vi "Vessel Blowout.vi"(7 "Blowtime(ms)":u32=5000, 9 "Delay(ms)":u32) -> ()   [LabVIEW 2019]
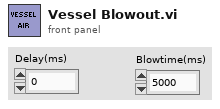
[diagram p1: front panel]
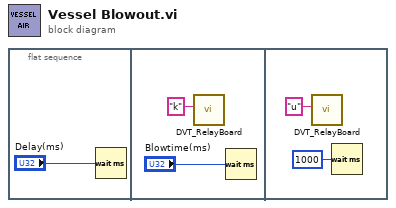
[diagram p0: block diagram]
diagram:
  n1 = flat-sequence {
    frame #0 {
      n2 = Wait (ms)(milliseconds to wait="Delay(ms)") -> ()  [unwired: 1 out]
    }
    frame #1 {
      n3 = call "DVT_RelayBoard.vi"("write buffer"="k") -> ()  [unwired: 3 in, 3 out]
      n4 = Wait (ms)(milliseconds to wait="Blowtime(ms)") -> ()  [unwired: 1 out]
    }
    frame #2 {
      n5 = call "DVT_RelayBoard.vi"("write buffer"="u") -> ()  [unwired: 3 in, 3 out]
      n6 = Wait (ms)(milliseconds to wait=u32 1000) -> ()  [unwired: 1 out]
    }
  }
